vi "checkForExistingControl.vi"(8 "error in (no error)":errorcluster, 9 "controlPath":path, 10 "libraryRef":refnum<vi>, 11 "Enumeration in":refnum<class "Enumeration.lvclass">) -> (0 "error out":errorcluster, 3 "Enumeration out":refnum<class "Enumeration.lvclass">)   [LabVIEW 2016, in "Enumeration.lvclass"]
uses:
  Enumeration.lvclass
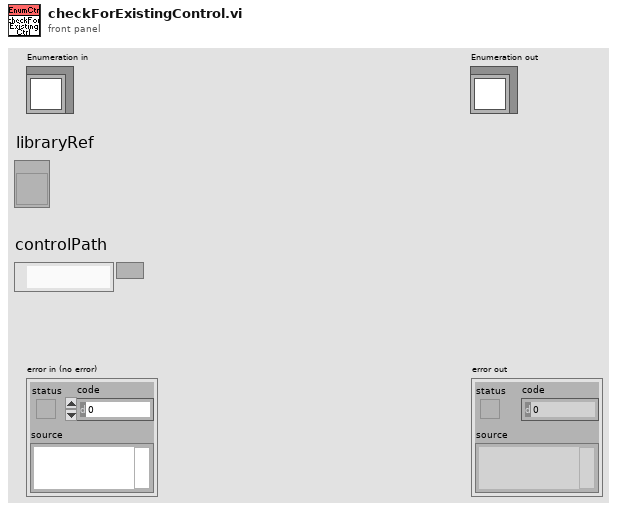
[diagram p1: front panel]
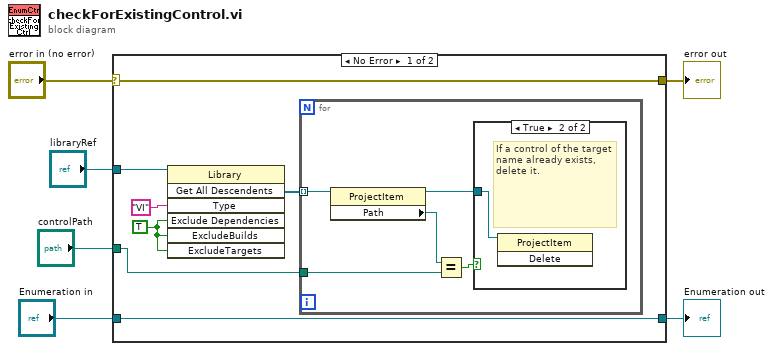
[diagram p0: block diagram]
diagram:
  n1 = case shown="No Error" "error in (no error)" {
    selector: "error in (no error)" -> [w12 w21]
    tunnel: [w12 w21] -> w5
    tunnel: [w13 w20] -> w3
    tunnel: "Enumeration in" -> [w13 w20]
    tunnel: "libraryRef" -> [w8 _]
    tunnel: "controlPath" -> [w7 _]
    frame No Error {
      w10 = TRUE ("ExcludeDependencies")
      n2 = invoke class="Library" method="Get All Descendents"(reference=w8, "Type"="VI", "Exclude Dependencies"=w10, "ExcludeBuilds"=w10, "ExcludeTargets"=w10) -> ("All Descendents"=w11:refnum<vi>[])  [unwired: 2 in, 6 out]
      n3 = for {
        tunnel: w11 -> [w18] mode=indexing
        tunnel: w7 -> [w16]
        n4 = property class="ProjectItem"(reference=w18) -> (reference out=w14:refnum<vi>, "Path"=w17:path)  [unwired: 1 in, 1 out]
        n5 = Equal?(x=w17, y=w16) -> (x = y?=w15:bool)
        n6 = case shown="True" w15 {
          tunnel: w14 -> [_ w19]
          frame False {
          }
          frame True {
            # "If a control of the target name already exists, delete it."
            n7 = invoke class="ProjectItem" method="Delete"(reference=w19) -> ()  [unwired: 2 in, 3 out]
          }
        }
      }
    }
    frame Error {
    }
  }
  "error out" <- w5
  "Enumeration out" <- w3
